vi "WPI_PotentiometerGetTestValue.vi"(8 "error in":errorcluster, 11 "PotDevRef":T1) -> (0 "error out":errorcluster, 2 "Test Value":dbl, 3 "PotDevRef":T1)   [LabVIEW 2017]
doc: "Returns the Normalized Value from the potentiometer. Normalization is the result of comparing the potentiometer return voltage to the 5 Volt Rail voltage of the controller that is used to power the potentiometer. This assures that the Normalized Value is from 0 to 1.\n\n\nThis software is licensed. Open the labview\\readme\\WPI Robotics Library Open Source License.txt file for more information."
uses:
  <vilib>/Rock Robotics/WPI/Potentiometer/WPI_PotentiometerDevRef.ctl
  <vilib>/Rock Robotics/SystemInterfaces/AI/FPGA_AIChannel.ctl
  <vilib>/Rock Robotics/WPI/AnalogChannel/WPI_AnalogChannelDevRef.ctl
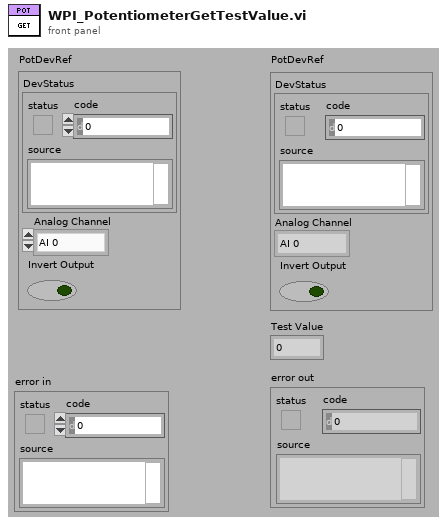
[diagram p1: front panel]
types:
  T1 = typedef "WPI_PotentiometerDevRef.ctl" = cluster{"DevStatus":errorcluster, "Analog Channel":T2, "Invert Output":bool}
  T2 = typedef "FPGA_AIChannel.ctl" = enum8{"AI 0", "AI 1", "AI 2", "AI 3", "AI MXP 0", "AI MXP 1", "AI MXP 2", "AI MXP 3", "Invalid"}
  T3 = typedef "WPI_AnalogChannelDevRef.ctl" = cluster{"DevStatus":errorcluster, "Analog Channel":T2}
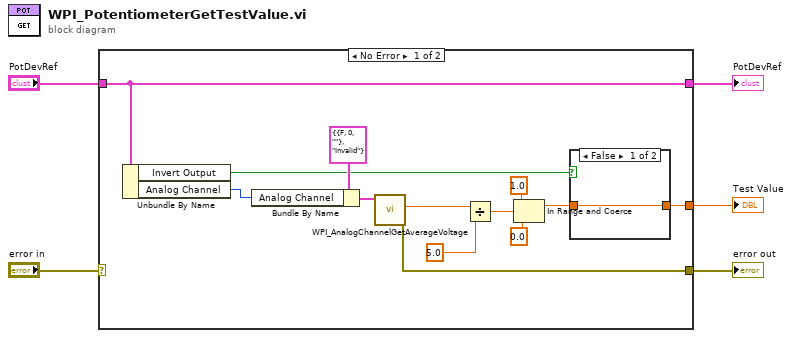
[diagram p0: block diagram]
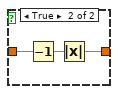
[diagram p2: hidden frame]
diagram:
  n1 = case shown="No Error" "error in" {
    selector: "error in" -> [_ w24]
    tunnel: "PotDevRef" -> [w14 w23]
    tunnel: [w6 w24] -> w4
    tunnel: [w9 _] -> w2
    tunnel: [w14 w23] -> w1
    frame No Error {
      n2 = Unbundle By Name(w14) -> ("Invert Output"=w8:bool, "Analog Channel"=w17:T2)
      n3 = Bundle By Name(cluster=T3 {"DevStatus"={"status"=FALSE, "code"=0, "source"=""}, "Analog Channel"=enum."Invalid"} ("AIDeviceRef"), "Analog Channel"=w17) -> (w16:T3)
      n4 = call <vilib>:"WPI_AnalogChannelGetAverageVoltage.vi"("AIDeviceRef"=w16) -> ("error out"=w6:errorcluster, "Voltage"=w15:dbl)  [unwired: 8 in, 1 out]
      n5 = Divide(x=w15, y=5.0 ("lower limit")) -> (x/y=w11:dbl)
      n6 = In Range and Coerce(upper limit=1.0, x=w11, lower limit=0.0) -> (coerced(x)=w10:dbl)  [unwired: 1 out]
      n7 = case shown="False" w8 {
        tunnel: w10 -> [w19 w21]
        tunnel: [w19 w20] -> w9
        frame False {
        }
        frame True {
          n8 = Decrement(x=w21) -> (x-1=w22:dbl)
          n9 = Absolute Value(x=w22) -> (abs(x)=w20:dbl)
        }
      }
    }
    frame Error {
    }
  }
  "PotDevRef" <- w1
  "Test Value" <- w2
  "error out" <- w4
